vi "Extract TSM DAQmx Single SSC.vi"(0 "DAQmx Tasks":refnum<k21>, 5 "Channel Lists":string, 7 "Per-Session Channel List":string) -> (4 "DAQ TSM SSC Multiple Out":T1)   [LabVIEW 2019]
uses:
  DAQmx/Pin Map/SSC DAQmx.ctl
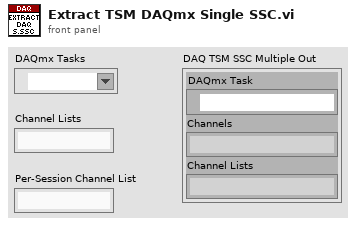
[diagram p1: front panel]
types:
  T1 = typedef "SSC DAQmx.ctl" = cluster{"DAQmx Task ":refnum<k21>, "Channels":string, "Channel Lists":string}
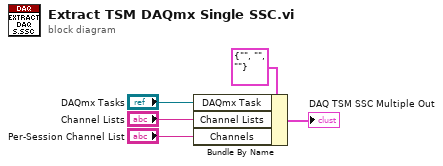
[diagram p0: block diagram]
diagram:
  n1 = Bundle By Name(cluster=T1 {"DAQmx Task "="", "Channels"="", "Channel Lists"=""} ("DAQmx SSC"), "DAQmx Task"="DAQmx Tasks", "Channel Lists"="Channel Lists", "Channels"="Per-Session Channel List") -> (→"DAQ TSM SSC Multiple Out":T1)
